vi "Prepare Subrequest.vi"(8 "error in (no error)":errorcluster, 11 "Multipart Parser in":refnum<class "Multipart Parser.lvclass">) -> (0 "error out":errorcluster, 3 "Multipart Parser out":refnum<class "Multipart Parser.lvclass">)   [LabVIEW 2020, in "HTTP Utils.lvlib" / "Multipart Parser.lvclass"]
uses:
  Multipart Parser.lvclass
  Multipart Parser.lvclass/Multipart Parser.ctl
  Request/Request.lvclass
  HTTP Utils.lvlib
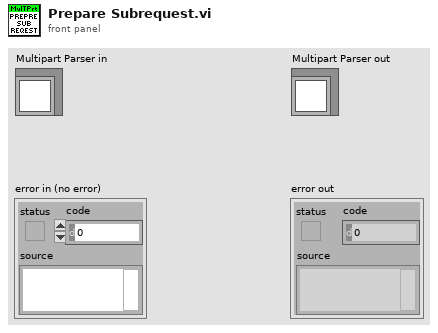
[diagram p1: front panel]
types:
  T1 = enum16{"open", "replace", "create", "open or create", "replace or create", "replace or create with confirmation"}
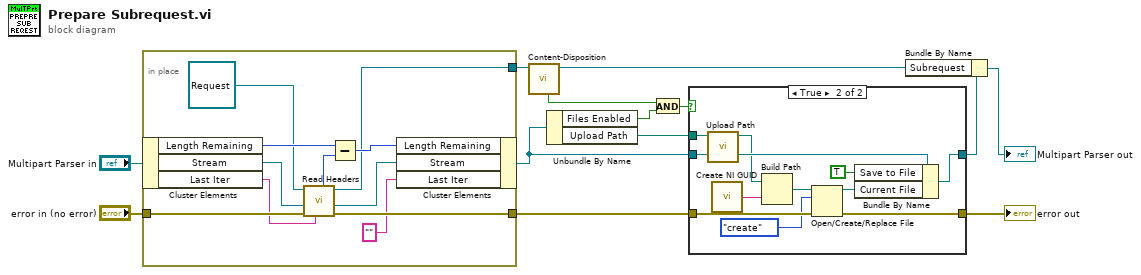
[diagram p0: block diagram]
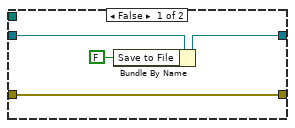
[diagram p2: hidden frame]
diagram:
  n1 = in-place {
    in-place-border: "error in (no error)" -> [w24]
    in-place-border: [w18] -> w11
    in-place-border: [w16] -> w10
    n2 = in-place-cluster #1("Multipart Parser in") -> ("Length Remaining"=w21:u64, "Stream"=w23:refnum<class "Stream.lvclass">, "Last Iter"=w15:string)
    n3 = call "Read Headers.vi"("Starting Buffer (None)"=w15, "error in (no error)"=w24, "Stream in"=w23, "Request in"=refnum<class "Request.lvclass"> refnum) -> ("error out"=w16:errorcluster, "Stream out"=w19:refnum<class "Stream.lvclass">, "Request out"=w18:refnum<class "Request.lvclass">, "Bytes"=w22:i32)  [unwired: 4 in]
    n4 = Subtract(x=w21, y=w22) -> (x-y=w20:u64)
    n5 = in-place-cluster #1("Length Remaining"=w20, "Stream"=w19, "Last Iter"="") -> (w9:refnum<class "Multipart Parser.lvclass">)
  }
  n6 = call "Content-Disposition.vi"("Request in"=w11) -> ("Request out"=w2:refnum<class "Request.lvclass">, "File?"=w7:bool)  [unwired: 6 in, 3 out]
  n7 = Unbundle By Name(w9) -> ("Files Enabled"=w8:bool, "Upload Path"=w5:path)
  n8 = And(x=w7, y=w8) -> (x .and. y?=w6:bool)
  n9 = case shown="True" w6 {
    tunnel: w10 -> [w25 w38]
    tunnel: w9 -> [w28 w37]
    tunnel: w5 -> [_ w39]
    tunnel: [w25 w31] -> w4
    tunnel: [w27 w29] -> w3
    frame False {
      n10 = Bundle By Name(cluster=w28, "Save to File"=FALSE) -> (w27:refnum<class "Multipart Parser.lvclass">)
    }
    frame True {
      n11 = call "Upload Path.vi"("Specified Path (Temp)"=w39) -> ("Upload Path"=w34:path)  [unwired: 10 in]
      n12 = call <vilib>:"Create NI GUID.vi"() -> ("NI GUID"=w35:string)
      n13 = Build Path(base path=w34, name or relative path=w35) -> (appended path=w33:path)
      n14 = Open/Create/Replace File(file path (use dialog)=w33, error in=w38, operation (0:open)=T1."create") -> (refnum out=w36:refnum<file>, error out=w31:errorcluster)  [unwired: 3 in, 1 out]
      n15 = Bundle By Name(cluster=w37, "Save to File"=TRUE, "Current File"=w36) -> (w29:refnum<class "Multipart Parser.lvclass">)
    }
  }
  "error out" <- w4
  n16 = Bundle By Name(cluster=w3, "Subrequest"=w2) -> (→"Multipart Parser out":refnum<class "Multipart Parser.lvclass">)
